vi "20190908_Move_Galvo_Mirror_with_buttons.vi"(11 "X set, Y set":dbl[](array[numeric])) -> ()   [LabVIEW 2015]
panel:
  in  "Control":enum16{"Go to set position", "Go to zero"}(ring)
  in  "?":bool
  in  "?":bool
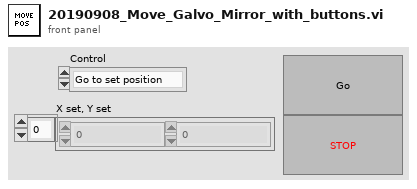
[diagram p1: front panel]
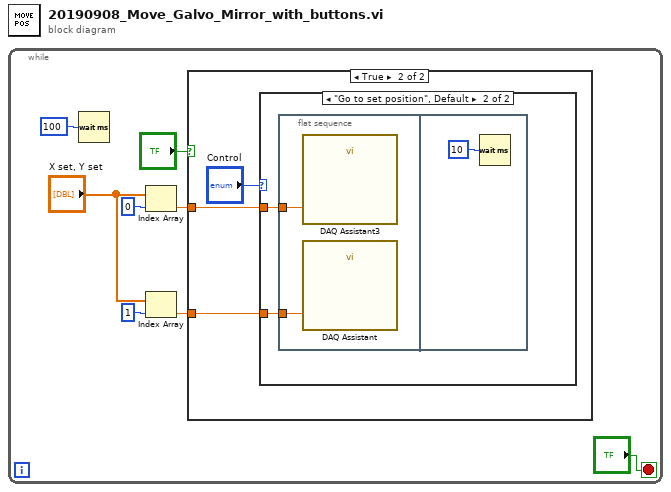
[diagram p0: block diagram]
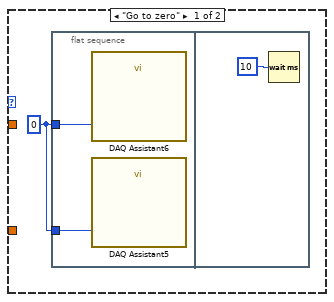
[diagram p3: hidden frame]
diagram:
  n1 = while {
    stop <- "?" stop-if-true
    n2 = Wait (ms)(milliseconds to wait=u32 100) -> ()  [unwired: 1 out]
    n3 = Index Array(array="X set, Y set", index=0) -> (element=w4:dbl)
    n4 = Index Array(array="X set, Y set", index=1) -> (element=w8:dbl)
    n5 = case shown="True" "?" {
      tunnel: w8 -> [_ w11]
      tunnel: w4 -> [_ w10]
      frame False {
      }
      frame True {
        n6 = case shown="\"Go to set position\", Default" "Control" {
          tunnel: w11 -> [_ w17]
          tunnel: w10 -> [_ w16]
          frame "Go to zero" {
            w12 = 0
            n7 = flat-sequence {
              tunnel: w12 -> [w14]
              tunnel: w12 -> [w13]
              frame #0 {
                n8 = call "DAQ Assistant6"("data"=w13) -> ()  [unwired: 17 in, 2 out]
                n9 = call "DAQ Assistant5"("data"=w14) -> ()  [unwired: 17 in, 2 out]
              }
              frame #1 {
                n10 = Wait (ms)(milliseconds to wait=u32 10) -> ()  [unwired: 1 out]
              }
            }
          }
          frame "Go to set position", Default {
            n11 = flat-sequence {
              tunnel: w17 -> [w19]
              tunnel: w16 -> [w18]
              frame #0 {
                n12 = call "DAQ Assistant3"("data"=w18) -> ()  [unwired: 17 in, 2 out]
                n13 = call "DAQ Assistant"("data"=w19) -> ()  [unwired: 17 in, 2 out]
              }
              frame #1 {
                n14 = Wait (ms)(milliseconds to wait=u32 10) -> ()  [unwired: 1 out]
              }
            }
          }
        }
      }
    }
  }
